vi "Sort Channel Reference 2D.vi"(10 "Cfg.AI":T1 {"References" items=["", "1", "2", "3"]; "Channel" min=1}) -> (2 "Channel Reference 2D":cluster{"Channel":i32, "Reference":i32}[][](array[cluster]))   [LabVIEW 2019, in "Instrument.Lockin.lvlib" / "Instrument.DAQ.lvclass"]
uses:
  Instrument.DAQ.lvclass
  Typedefs/AI.Channel--Cluster.ctl
  Typedefs/AI.Channel--Cluster--Array.ctl
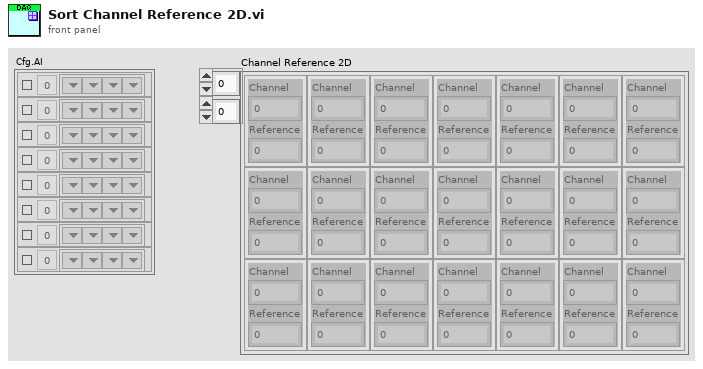
[diagram p1: front panel]
types:
  T1 = typedef "Instrument.Lockin.lvlib/Instrument.DAQ.lvclass/AI.Channel--Cluster--Array.ctl" = T2[]
  T2 = typedef "Instrument.Lockin.lvlib/Instrument.DAQ.lvclass/AI.Channel--Cluster.ctl" = cluster{"Enable?":bool, "Channel":i32, "References":i32[]}
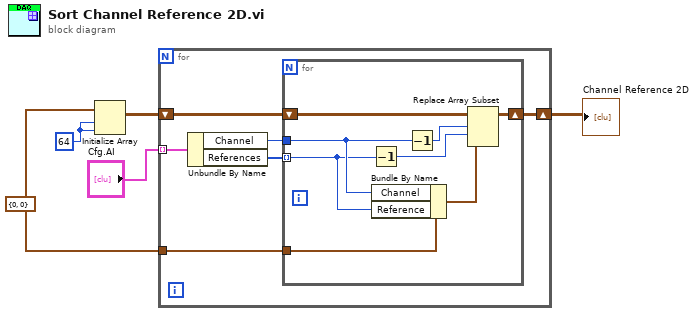
[diagram p0: block diagram]
diagram:
  w1 = cluster{"Channel":i32, "Reference":i32} {"Channel"=0, "Reference"=0}
  w4 = 64 ("dimension size")
  n1 = Initialize Array(w1, w4, w4) -> (w3:cluster{"Channel":i32, "Reference":i32}[][])
  n2 = for {
    tunnel: "Cfg.AI" -> [w11] mode=indexing
    shift-right: [w9] -> w2
    shift-left: w3 -> [w8]
    tunnel: w1 -> [w6]
    n3 = Unbundle By Name(w11) -> ("Channel"=w7:i32, "References"=w10:i32[])
    n4 = for {
      tunnel: w10 -> [w13] mode=indexing
      shift-right: [w18] -> w9
      shift-left: w8 -> [w19]
      tunnel: w7 -> [w14]
      tunnel: w6 -> [w15]
      n5 = Decrement(x=w13) -> (x-1=w16:i32)
      n6 = Bundle By Name(cluster=w15, "Channel"=w14, "Reference"=w13) -> (w12:cluster{"Channel":i32, "Reference":i32})
      n7 = Decrement(x=w14) -> (x-1=w17:i32)
      n8 = Replace Array Subset(array=w19, new element=w12, index (row)=w17, index (col)=w16) -> (w18:cluster{"Channel":i32, "Reference":i32}[][])
    }
  }
  "Channel Reference 2D" <- w2
